vi "Open_BP4610.vi"(8 "error in (no error)":errorcluster, 11 "VISAsession":refnum<visa-resource-name>) -> (0 "error out":errorcluster, 3 "CopyVISAsession":refnum<visa-resource-name>)   [LabVIEW 2019]
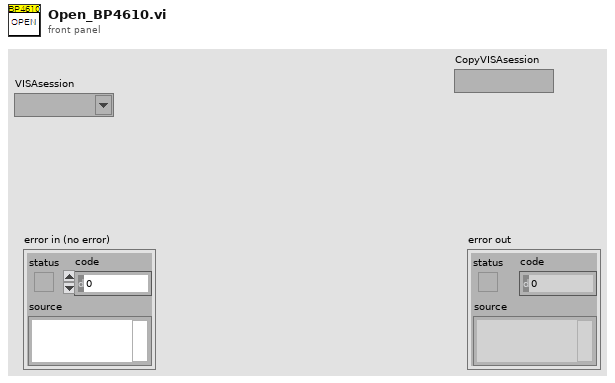
[diagram p1: front panel]
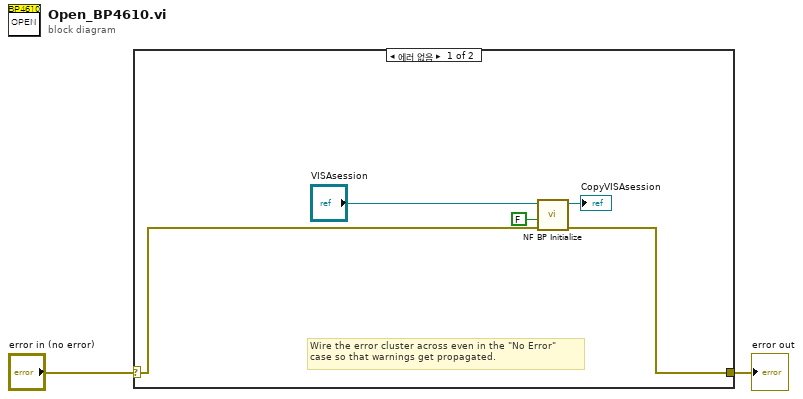
[diagram p0: block diagram]
diagram:
  n1 = case shown="에러 없음" "error in (no error)" {
    selector: "error in (no error)" -> [w6 w8]
    tunnel: [w5 w8] -> w1
    frame No Error {
      # "Wire the error cluster across even in the \"No Error\"\ncase so that warnings get propagated."
      n2 = call <instrlib>:"NF BP Initialize.vi"("error in (no error)"=w6, "Reset(T)"=FALSE ("Read"), "VISAsession"="VISAsession") -> ("error out"=w5:errorcluster, "CopyVISAsession"=→"CopyVISAsession":refnum<visa-resource-name>)  [unwired: 6 in, 1 out]
    }
    frame Error {
    }
  }
  "error out" <- w1
